vi "LidarTest.vi"() -> ()   [LabVIEW 2017]
panel:
  out "size(s)":i32
  in  "stop":bool
  out "XY Graph":cluster{dbl[], dbl[]}(graph)
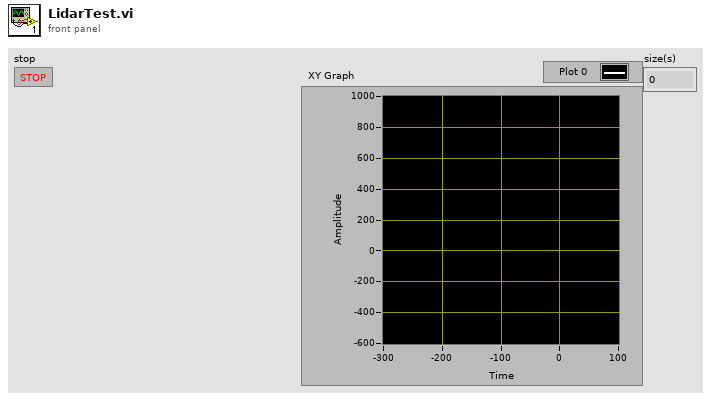
[diagram p1: front panel]
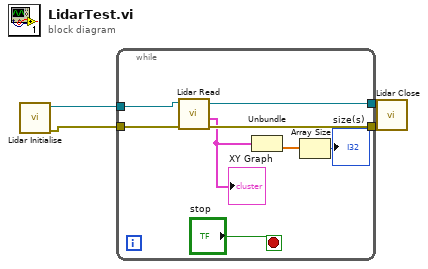
[diagram p0: block diagram]
diagram:
  n1 = call "Lidar Initialise.vi"() -> ("error out"=w3:errorcluster, "VISA resource name out"=w4:refnum<visa-resource-name>)  [unwired: 10 in]
  n2 = while {
    tunnel: w4 -> [w12]
    tunnel: w3 -> [w11]
    tunnel: [w10] -> w2
    tunnel: [w9] -> w1
    stop <- "stop" stop-if-true
    n3 = call "Lidar Read.vi"("error in (no error)"=w11, "VISA resource name"=w12) -> ("error out"=w9:errorcluster, "Visual Out"=w7:cluster{dbl[], dbl[]}, "VISA resource name out"=w10:refnum<visa-resource-name>)  [unwired: 2 in, 4 out]
    "XY Graph" <- w7
    n4 = Unbundle(w7) -> (w6:dbl[])  [unwired: 1 out]
    n5 = Array Size(array=w6) -> (size(s)=→"size(s)":i32)
  }
  n6 = call "Lidar Close.vi"("error in (no error)"=w1, "VISA resource name"=w2) -> ()  [unwired: 9 in, 1 out]
